vi "CleanUp.vi"(8 "Error In":errorcluster, 11 "Object in":refnum<class "Board Game.lvclass">) -> (0 "Error Out":errorcluster, 3 "object out":refnum<class "Board Game.lvclass">)   [LabVIEW 2021, in "Board Game.lvclass"]
uses:
  Board Game.lvclass
  Board Game.lvclass/Board Game.ctl
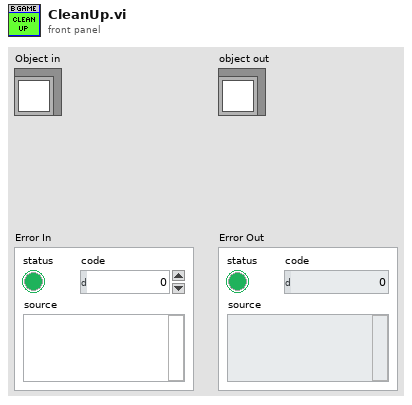
[diagram p1: front panel]
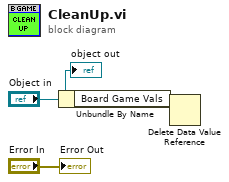
[diagram p0: block diagram]
diagram:
  n1 = Unbundle By Name("Object in") -> ("Board Game Vals"=w2:refnum<data-value>)
  n2 = Delete Data Value Reference(data value reference=w2) -> ()  [unwired: 1 in, 2 out]
  "Error Out" <- "Error In"
  "object out" <- "Object in"
